vi "Override Transfer Groups.vi"(8 "error in (no error)":errorcluster, 10 "All Transfers":refnum<class "Transfer Group.lvclass">[](array[class]), 11 "Mock Framework in":refnum<class "Mock Framework.lvclass">) -> (0 "error out":errorcluster, 3 "Mock Framework out":refnum<class "Mock Framework.lvclass">)   [LabVIEW 2017, in "Mock Framework.lvclass"]
uses:
  Mock Framework.lvclass
  C:/github/data-sharing-framework/Data Sharing Framework Core/Engine/Classes/Framework/Framework.lvclass
  Engine/Classes/Transfer Group/Transfer Group.lvclass
  Engine/Classes/Framework/Framework.lvclass/Framework.ctl
  Engine/Classes/Framework/Framework.lvclass
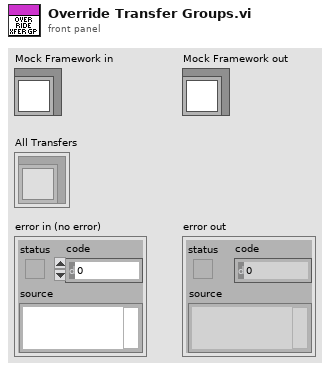
[diagram p1: front panel]
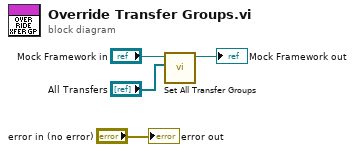
[diagram p0: block diagram]
diagram:
  n1 = call "Set All Transfer Groups.vi"("All Transfer Groups"="All Transfers", "Framework in"="Mock Framework in") -> ("Framework out"=→"Mock Framework out":refnum<class "Mock Framework.lvclass">)  [unwired: 9 in]
  "error out" <- "error in (no error)"
